vi "NumBoolsTrue.vi"(10 "# True":i32, 11 "Signals In":bool[](array[boolean])) -> (2 "Actual Number":i32, 3 "Number Met?":bool)   [LabVIEW 2017]
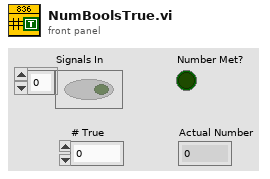
[diagram p1: front panel]
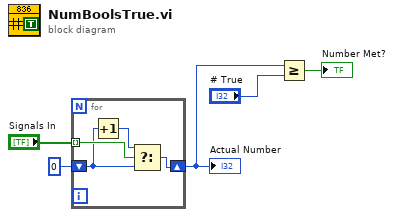
[diagram p0: block diagram]
diagram:
  n1 = for {
    tunnel: "Signals In" -> [w9] mode=indexing
    shift-right: [w6] -> w3
    shift-left: 0 -> [w7]
    n2 = Increment(x=w7) -> (x+1=w8:i32)
    n3 = Select(t=w8, s=w9, f=w7) -> (s? t:f=w6:i32)
  }
  "Actual Number" <- w3
  n4 = Greater Or Equal?(x=w3, y="# True") -> (x >= y?=→"Number Met?":bool)
